vi "Sensitivity.vi"(8 "Sensitivity":dbl, 9 "Low":dbl, 10 "High":dbl, 11 "Signal":dbl) -> (2 "Output":dbl)   [LabVIEW 2017]
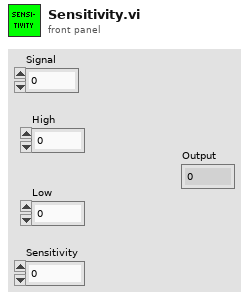
[diagram p1: front panel]
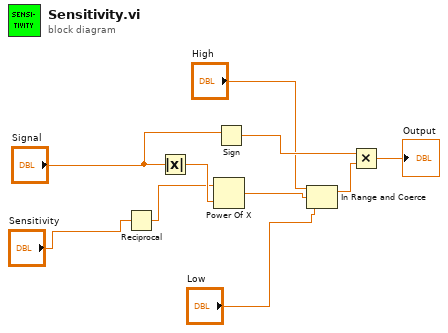
[diagram p0: block diagram]
diagram:
  n1 = Reciprocal(x="Sensitivity") -> (1/x=w3:dbl)
  n2 = Absolute Value(x="Signal") -> (abs(x)=w10:dbl)
  n3 = Power Of X(1:w10, 2:w3) -> (0:w8:dbl)
  n4 = Sign(1:"Signal") -> (0:w9:dbl)
  n5 = In Range and Coerce(upper limit="High", x=w8, lower limit="Low") -> (coerced(x)=w7:dbl)  [unwired: 1 out]
  n6 = Multiply(x=w9, y=w7) -> (x*y=→"Output":dbl)
